vi "Ocitavanje.vi"() -> ()   [LabVIEW 2014]
panel:
  out "error out":errorcluster
  in  "error in (no error)":errorcluster
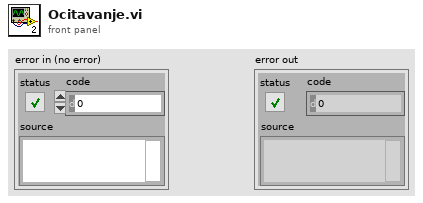
[diagram p1: front panel]
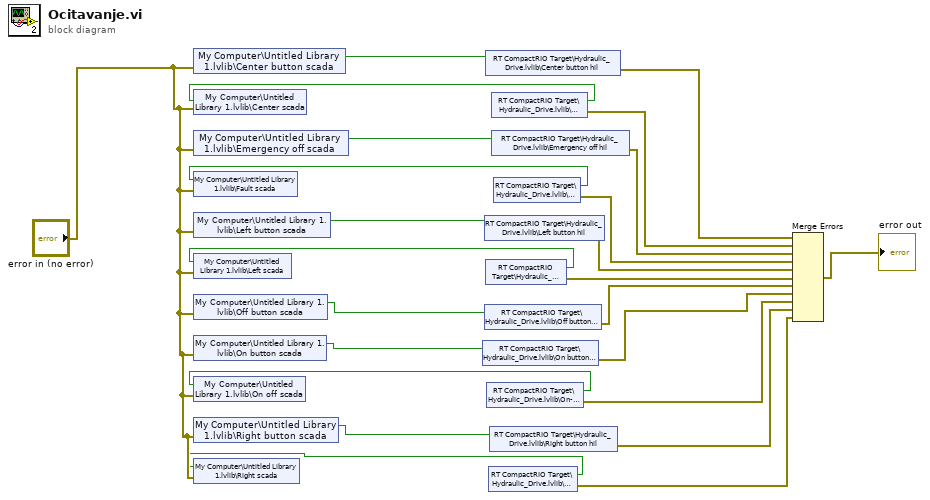
[diagram p0: block diagram]
diagram:
  n1 = shared-variable "My Computer\\Untitled Library 1.lvlib\\Center button scada"(error in="error in (no error)") -> (w23:bool)  [unwired: 1 out]
  n2 = shared-variable "My Computer\\Untitled Library 1.lvlib\\Emergency off scada"(error in="error in (no error)") -> (w21:bool)  [unwired: 1 out]
  n3 = shared-variable "My Computer\\Untitled Library 1.lvlib\\Left button scada"(error in="error in (no error)") -> (w19:bool)  [unwired: 1 out]
  n4 = shared-variable "My Computer\\Untitled Library 1.lvlib\\Off button scada"(error in="error in (no error)") -> (w17:bool)  [unwired: 1 out]
  n5 = shared-variable "My Computer\\Untitled Library 1.lvlib\\On button scada"(error in="error in (no error)") -> (w16:bool)  [unwired: 1 out]
  n6 = shared-variable "My Computer\\Untitled Library 1.lvlib\\Right button scada"(error in="error in (no error)") -> (w14:bool)  [unwired: 1 out]
  n7 = shared-variable "RT CompactRIO Target\\Hydraulic_Drive.lvlib\\On button hil"(w16) -> (error out=w4:errorcluster)  [unwired: 1 in]
  n8 = shared-variable "RT CompactRIO Target\\Hydraulic_Drive.lvlib\\Left button hil"(w19) -> (error out=w7:errorcluster)  [unwired: 1 in]
  n9 = shared-variable "RT CompactRIO Target\\Hydraulic_Drive.lvlib\\Off button hil"(w17) -> (error out=w5:errorcluster)  [unwired: 1 in]
  n10 = shared-variable "RT CompactRIO Target\\Hydraulic_Drive.lvlib\\Center button hil"(w23) -> (error out=w11:errorcluster)  [unwired: 1 in]
  n11 = shared-variable "RT CompactRIO Target\\Hydraulic_Drive.lvlib\\Left hil"() -> (w18:bool, error out=w6:errorcluster)  [unwired: 1 in]
  n12 = shared-variable "My Computer\\Untitled Library 1.lvlib\\Left scada"(w18, error in="error in (no error)") -> ()  [unwired: 1 out]
  n13 = shared-variable "RT CompactRIO Target\\Hydraulic_Drive.lvlib\\On-off hil"() -> (w15:bool, error out=w3:errorcluster)  [unwired: 1 in]
  n14 = shared-variable "My Computer\\Untitled Library 1.lvlib\\On off scada"(w15, error in="error in (no error)") -> ()  [unwired: 1 out]
  n15 = shared-variable "RT CompactRIO Target\\Hydraulic_Drive.lvlib\\Right hil"() -> (w13:bool, error out=w1:errorcluster)  [unwired: 1 in]
  n16 = shared-variable "My Computer\\Untitled Library 1.lvlib\\Right scada"(w13, error in="error in (no error)") -> ()  [unwired: 1 out]
  n17 = shared-variable "RT CompactRIO Target\\Hydraulic_Drive.lvlib\\Right button hil"(w14) -> (error out=w2:errorcluster)  [unwired: 1 in]
  n18 = shared-variable "RT CompactRIO Target\\Hydraulic_Drive.lvlib\\Center hil"() -> (w22:bool, error out=w10:errorcluster)  [unwired: 1 in]
  n19 = shared-variable "My Computer\\Untitled Library 1.lvlib\\Center scada"(w22, error in="error in (no error)") -> ()  [unwired: 1 out]
  n20 = shared-variable "RT CompactRIO Target\\Hydraulic_Drive.lvlib\\Emergency off hil"(w21) -> (error out=w9:errorcluster)  [unwired: 1 in]
  n21 = shared-variable "RT CompactRIO Target\\Hydraulic_Drive.lvlib\\Fault hil"() -> (w20:bool, error out=w8:errorcluster)  [unwired: 1 in]
  n22 = shared-variable "My Computer\\Untitled Library 1.lvlib\\Fault scada"(w20, error in="error in (no error)") -> ()  [unwired: 1 out]
  n23 = Merge Errors(w11, w10, w9, w8, w7, w6, w5, w4, w3, w2, w1) -> (→"error out":errorcluster)
